vi "Test CameraTool Get Fiducial Manual.vi"() -> ()   [LabVIEW 2011]
uses:
  Config Manager Class/Type Definitions/Camera Enum.ctl
  Gantry Class/Gantry Class.lvclass
  Vec3d Class/Vec3d Class.lvclass
panel:
  out "Current Position":cluster{"X":dbl, "Y":dbl, "Z":dbl}
  in  "stop":bool
  out "preview":T1(plugin-control)
  in  "Control Scheme":enum16{"MPG Control", "Mouse Control"}(ring)
  out "error out":errorcluster
  in  "Config Folder":path=path "C:/Users/Husker/Desktop/gantry/Config"
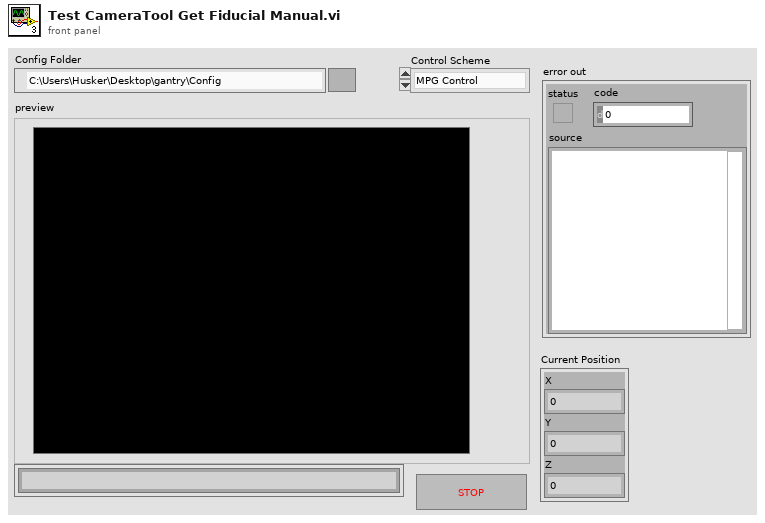
[diagram p1: front panel]
types:
  T1 = typedef "IMAQ Image.ctl" = refnum<image>
  T2 = typedef "Camera Enum.ctl" = enum16{"GANTRY HEAD", "NEEDLE CALIBRATION X", "NEEDLE CALIBRATION Y"}
  T3 = typedef "Physical Image.ctl" = cluster{"Image Position":refnum<class "Vec3d Class.lvclass">, "Image Reference":T1, "Field of View":cluster{"x(mm)":dbl, "y(mm)":dbl}}
  T4 = typedef "LVPoint32TypeDef.ctl" = cluster{"Horizontal":i32, "Vertical":i32}
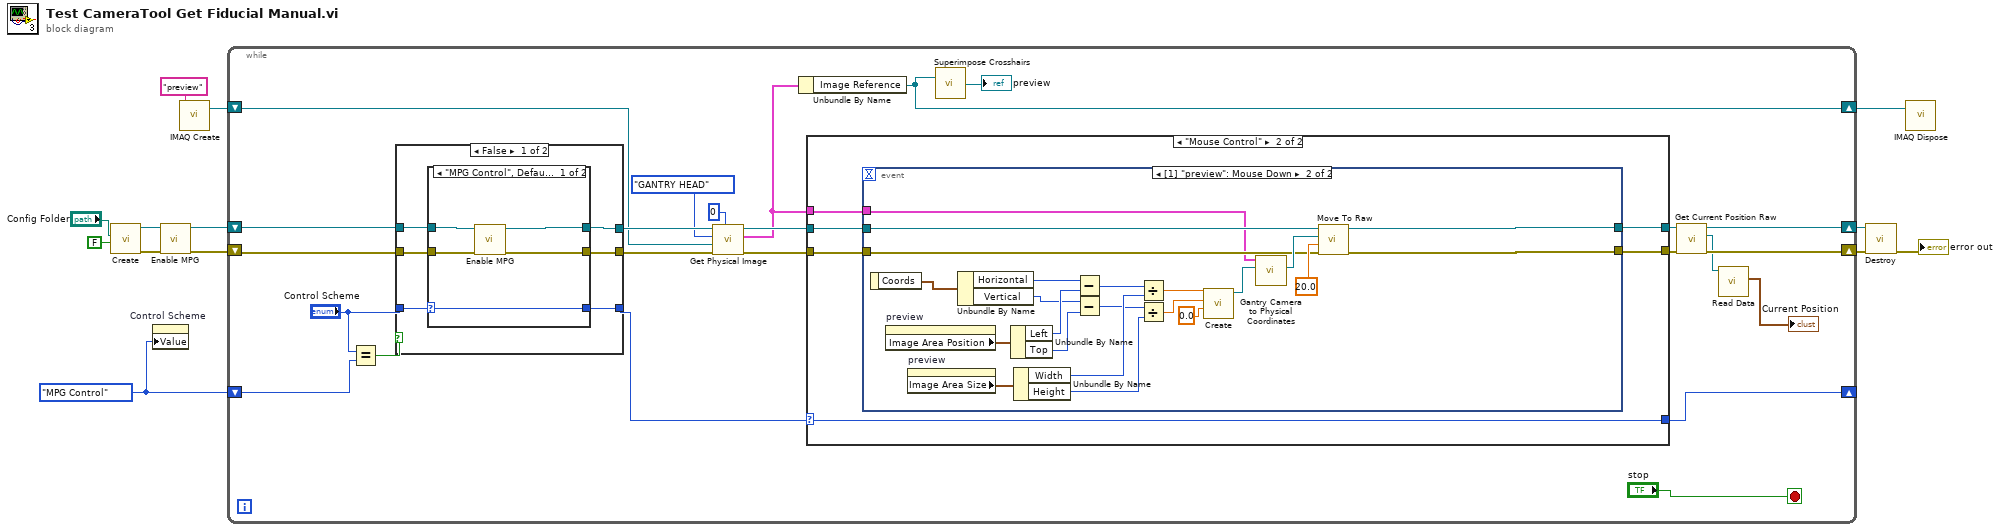
[diagram p0: block diagram]
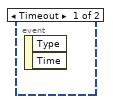
[diagram p3: hidden frame]
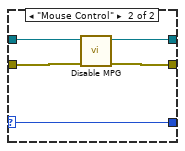
[diagram p4: hidden frame]
diagram:
  w3 = enum16{"MPG Control", "Mouse Control"}."MPG Control" ("Control Scheme 2")
  n1 = call "Create.vi"("HOME?"=FALSE, "Config Folder"="Config Folder") -> ("error out"=w7:errorcluster, "Gantry out"=w9:refnum<class "Gantry Class.lvclass">)  [unwired: 8 in]
  n2 = property on="Control Scheme" class="Enum (strict)"("Value"=w3) -> ()  [unwired: 2 in, 2 out]
  n3 = call-dynamic "Enable MPG.vi"("error in"=w7, "Gantry in"=w9) -> ("error out"=w5:errorcluster, "Gantry out"=w8:refnum<class "Gantry Class.lvclass">)  [unwired: 8 in]
  n4 = call "IMAQ Create"("Image Name"="preview") -> ("New Image"=w6:T1)  [unwired: 4 in, 1 out]
  n5 = while {
    shift-right: [w28] -> _
    shift-left: w3 -> [w37]
    shift-right: [w17] -> w4
    shift-left: w6 -> [w30]
    shift-right: [w22] -> w2
    shift-left: w8 -> [w35]
    shift-right: [w20] -> w1
    shift-left: w5 -> [w33]
    stop <- "stop" stop-if-true
    n6 = Equal?(x="Control Scheme", y=w37) -> (x = y?=w36:bool)
    n7 = case shown="False" w36 {
      tunnel: w35 -> [w73 w87]
      tunnel: [w72 w87] -> w31
      tunnel: "Control Scheme" -> [w74 w85]
      tunnel: w33 -> [w71 w86]
      tunnel: [w70 w86] -> w32
      tunnel: [w69 w85] -> w29
      frame False {
        n8 = case shown="\"MPG Control\", Default" w74 {
          selector: w74 -> [w75 w80]
          tunnel: w73 -> [w79 w84]
          tunnel: [w78 w83] -> w72
          tunnel: w71 -> [w77 w82]
          tunnel: [w76 w81] -> w70
          tunnel: [w75 w80] -> w69
          frame "MPG Control", Default {
            n9 = call-dynamic "Enable MPG.vi"("error in"=w77, "Gantry in"=w79) -> ("error out"=w76:errorcluster, "Gantry out"=w78:refnum<class "Gantry Class.lvclass">)  [unwired: 8 in]
          }
          frame "Mouse Control" {
            n10 = call-dynamic "Disable MPG.vi"("error in"=w82, "Gantry in"=w84) -> ("error out"=w81:errorcluster, "Gantry out"=w83:refnum<class "Gantry Class.lvclass">)  [unwired: 8 in]
          }
        }
      }
      frame True {
      }
    }
    n11 = call-dynamic "Get Physical Image.vi"("Delay(milliseconds)"=0, "error in"=w32, "Image In"=w30, "Camera Name"=Camera_Enum."GANTRY HEAD", "Gantry in"=w31) -> ("error out"=w26:errorcluster, "Physical Image"=w16:T3, "Gantry out"=w27:refnum<class "Gantry Class.lvclass">)  [unwired: 4 in]
    n12 = Unbundle By Name(w16) -> ("Image Reference"=w17:T1)
    n13 = case shown="\"Mouse Control\"" w29 {
      selector: w29 -> [w40 w46]
      tunnel: [w40 w46] -> w28
      tunnel: w27 -> [w39 w45]
      tunnel: [w39 w44] -> w23
      tunnel: w26 -> [w38 w43]
      tunnel: [w38 w42] -> w21
      tunnel: w16 -> [_ w41]
      frame "MPG Control", Default {
      }
      frame "Mouse Control" {
        n14 = event shown="[1] \"preview\": Mouse Down" {
          selector: _ -> [_ _]
          dyn-events: _ -> [_ _]
          timeout: _ -> [_ _]
          tunnel: w45 -> [_ w49]
          tunnel: [_ w63] -> w44
          tunnel: w43 -> [_ w48]
          tunnel: [_ w62] -> w42
          tunnel: w41 -> [_ w47]
          event Timeout {
            n15 = event-data() -> ()  [unwired: 1 in, 2 out]
          }
          event "preview": Mouse Down {
            n16 = event-data() -> ("Coords"=w61:T4)  [unwired: 1 in]
            n17 = property on="preview" class="ImageControl"() -> ("Image Area Position"=w60:cluster{"Left":i32, "Top":i32})  [unwired: 2 in, 2 out]
            n18 = property on="preview" class="ImageControl"() -> ("Image Area Size"=w55:cluster{"Width":u32, "Height":u32})  [unwired: 2 in, 2 out]
            n19 = Unbundle By Name(w61) -> ("Horizontal"=w59:i32, "Vertical"=w57:i32)
            n20 = Unbundle By Name(w60) -> ("Left"=w58:i32, "Top"=w56:i32)
            n21 = Unbundle By Name(w55) -> ("Width"=w53:u32, "Height"=w51:u32)
            n22 = Subtract(x=w59, y=w58) -> (x-y=w68:i32)
            n23 = Subtract(x=w57, y=w56) -> (x-y=w52:i32)
            n24 = Divide(x=w68, y=w53) -> (x/y=w54:dbl)
            n25 = Divide(x=w52, y=w51) -> (x/y=w50:dbl)
            n26 = call "Create.vi"("Z"=0.0, "Y"=w50, "X"=w54) -> ("Vec3d Class out"=w66:refnum<class "Vec3d Class.lvclass">)  [unwired: 7 in, 1 out]
            n27 = call "Gantry Camera to Physical Coordinates.vi"("Image Coordinate"=w66, "Physical Image"=w47) -> ("Global Coordinate"=w65:refnum<class "Vec3d Class.lvclass">)  [unwired: 7 in, 2 out]
            n28 = call-dynamic "Move To Raw.vi"("error in"=w48, "Speed"=20.0, "Destination"=w65, "Gantry in"=w49) -> ("error out"=w62:errorcluster, "Gantry out"=w63:refnum<class "Gantry Class.lvclass">)  [unwired: 6 in]
          }
        }
      }
    }
    n29 = call "Superimpose Crosshairs.vi"("Refnum in"=w17) -> ("Refnum out"=→"preview":T1)  [unwired: 1 in]
    n30 = call-dynamic "Get Current Position Raw.vi"("error in"=w21, "Gantry in"=w23) -> ("error out"=w20:errorcluster, "Vec3d Class out"=w19:refnum<class "Vec3d Class.lvclass">, "Gantry out"=w22:refnum<class "Gantry Class.lvclass">)  [unwired: 7 in]
    n31 = call-dynamic "Read Data.vi"("Vec3d Class in"=w19) -> ("Data"=→"Current Position":cluster{"X":dbl, "Y":dbl, "Z":dbl})  [unwired: 8 in, 2 out]
  }
  n32 = call "Destroy.vi"("error in"=w1, "Gantry Class in"=w2) -> ("error out"=→"error out":errorcluster)  [unwired: 9 in]
  n33 = call "IMAQ Dispose"("Image"=w4) -> ()  [unwired: 5 in, 1 out]
